vi "FreeMemInfo.vi"(7 "error in (no error)":errorcluster) -> (0 "error out":errorcluster, 1 "PhysicalFreeSpace":dbl format="%.2f", 2 "PhysicalSpace":dbl format="%.2f")   [LabVIEW 2015, in "ESLSCDLL.lvlib"]
uses:
  ESLSCDLL.lvlib
  Globals.vi
panel:
  # "MB"
  # "MB"
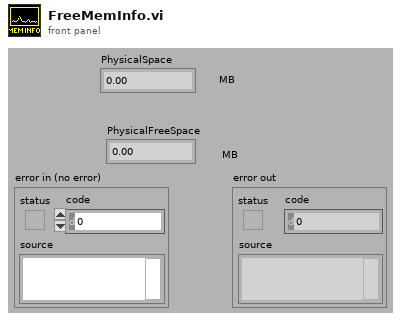
[diagram p1: front panel]
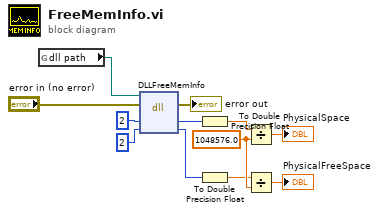
[diagram p0: block diagram]
diagram:
  w10 = 1048576.0
  n1 = global read "Globals.vi" "dll path"() -> (w1:path)
  n2 = dll-call lib="C:/ENTW/PCIE/LV64/board.vis/ESLSCDLL.dll" fn="DLLFreeMemInfo"(path in=w1, error in="error in (no error)", "memory_all"=u64 2, "memory_free"=u64 2) -> (error out=→"error out":errorcluster, "memory_all"=w4:u64, "memory_free"=w5:u64)  [unwired: 2 in, 1 out]
  n3 = To Double Precision Float(number=w4) -> (double precision float=w7:dbl)
  n4 = To Double Precision Float(number=w5) -> (double precision float=w6:dbl)
  n5 = Divide(x=w7, y=w10) -> (x/y=→"PhysicalSpace":dbl)
  n6 = Divide(x=w6, y=w10) -> (x/y=→"PhysicalFreeSpace":dbl)
